vi "FD7C8LXI697RGWP.vi"() -> ()   [LabVIEW 2017]
uses:
  <vilib>/Instr/_visa.llb/VISA Configure Serial Port (Instr).vi
panel:
  out "Available?":bool
  in  "COM Port":refnum<visa-resource-name>
  in  "Baud Rate":u32=9600
  out "Num Inds":dbl
  in  "Stop Button":bool
  in  "Turn Off":bool
  in  "Turn On":bool
  out "Waveform Chart":dbl(graph)
  out "Thermometer":dbl(slide) scale=0.0..100.0
  # "LM35"
  # "USB Control"
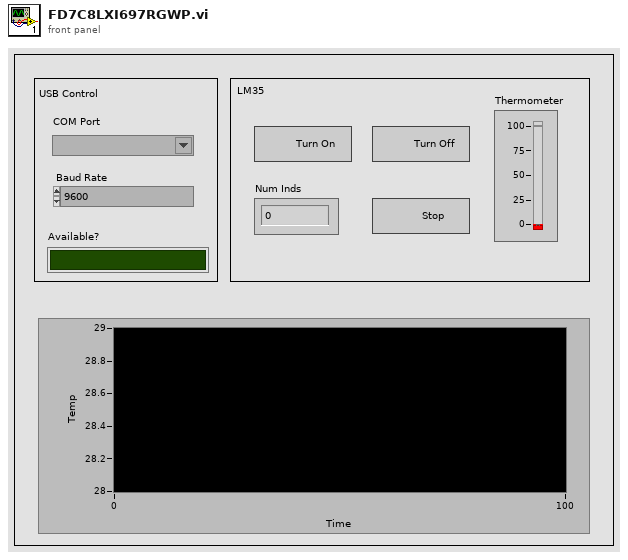
[diagram p1: front panel]
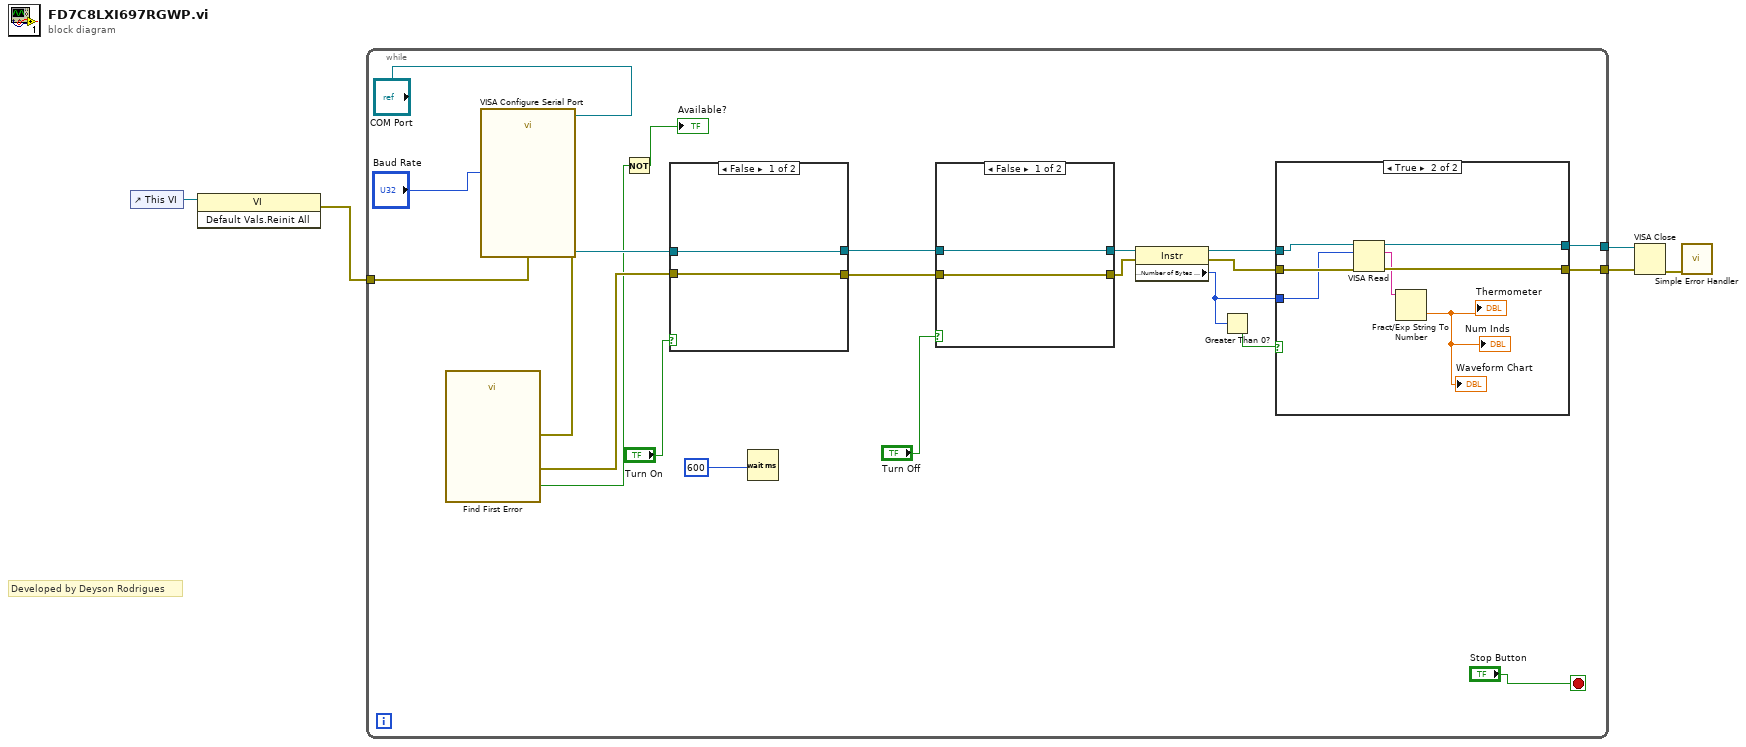
[diagram p0: block diagram]
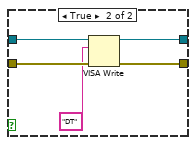
[diagram p3: hidden frame]
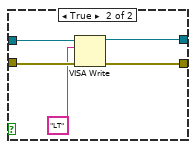
[diagram p4: hidden frame]
diagram:
  # "Developed by Deyson Rodrigues"
  n1 = control-ref of="This VI"() -> (w1:refnum<vi>)
  n2 = invoke class="VI" method="Default Vals.Reinit All"(reference=w1) -> (error out=w2:errorcluster)  [unwired: 2 in, 2 out]
  n3 = while {
    tunnel: [w20] -> w4
    tunnel: [w19] -> w5
    tunnel: w2 -> [w6]
    stop <- "Stop Button" stop-if-true
    n4 = call-poly "VISA Configure Serial Port"("VISA resource name"="COM Port", "baud rate (9600)"="Baud Rate", "error in (no error)"=w6) -> ("VISA resource name out"=w11:refnum<visa-resource-name>, "error out"=w9:errorcluster)  [unwired: 11 in]
    n5 = call <vilib>:"Find First Error.vi"("error in (no error)"=w9) -> ("error out"=w10:errorcluster, "error?"=w8:bool)  [unwired: 3 in]
    n6 = Not(x=w8) -> (.not. x?=→"Available?":bool)
    n7 = case shown="False" "Turn On" {
      tunnel: [w45 w50] -> w27
      tunnel: [w44 w49] -> w26
      tunnel: w11 -> [w45 w48]
      tunnel: w10 -> [w44 w47]
      frame False {
      }
      frame True {
        n8 = VISA Write(VISA resource name=w48, write buffer="LT", error in (no error)=w47) -> (VISA resource name out=w50:refnum<visa-resource-name>, error out=w49:errorcluster)  [unwired: 1 out]
      }
    }
    n9 = Wait (ms)(milliseconds to wait=u32 600 ("millisecond timer value")) -> ()  [unwired: 1 out]
    n10 = case shown="False" "Turn Off" {
      tunnel: w27 -> [w38 w43]
      tunnel: w26 -> [w37 w42]
      tunnel: [w37 w41] -> w24
      tunnel: [w38 w40] -> w25
      frame False {
      }
      frame True {
        n11 = VISA Write(VISA resource name=w43, write buffer="DT", error in (no error)=w42) -> (VISA resource name out=w40:refnum<visa-resource-name>, error out=w41:errorcluster)  [unwired: 1 out]
      }
    }
    n12 = property class="Instr"(reference=w25, error in=w24) -> (reference out=w21:refnum<visa-resource-name>, error out=w22:errorcluster, "Serial Settings:Number of Bytes at Serial Port"=w18:u32)
    n13 = Greater Than 0?(x=w18) -> (x > 0?=w23:bool)
    n14 = case shown="True" w23 {
      tunnel: w21 -> [w29 w36]
      tunnel: w22 -> [w28 w34]
      tunnel: [w29 w35] -> w20
      tunnel: [w28 w33] -> w19
      tunnel: w18 -> [_ w32]
      frame False {
      }
      frame True {
        n15 = VISA Read(VISA resource name=w36, byte count=w32, error in (no error)=w34) -> (VISA resource name out=w35:refnum<visa-resource-name>, read buffer=w31:string, error out=w33:errorcluster)  [unwired: 1 out]
        n16 = Fract/Exp String To Number(string=w31) -> (number=→"Thermometer" →"Num Inds" →"Waveform Chart":dbl)  [unwired: 3 in, 1 out]
      }
    }
  }
  n17 = VISA Close(VISA resource name=w4, error in (no error)=w5) -> (error out=w3:errorcluster)
  n18 = call <vilib>:"Simple Error Handler.vi"("error in (no error)"=w3) -> ()  [unwired: 4 in, 5 out]
